vi "send response.vi"(6 "udp message":string, 7 "connection ID out":refnum<k16>, 8 "error in (no error)":errorcluster, 9 "port":u16, 10 "address":u32, 11 "command_parser in":refnum<class "command_parser.lvclass">) -> (0 "error out":errorcluster, 3 "command_parser out":refnum<class "command_parser.lvclass">)   [LabVIEW 2025, in "command_parser.lvlib" / "command_parser.lvclass"]
uses:
  command_parser.lvclass
  Applications/National Instruments/LabVIEW 2025 64-bit/vi.lib/ActorFramework/Actor/Actor.lvclass
  command_parser.lvclass/command_parser.ctl
  Send Notification Messages/send response Msg/send response Msg.lvclass/send response Msg.ctl
  <vilib>/ActorFramework/Message Enqueuer/Message Enqueuer.lvclass/Message Enqueuer.ctl
  <vilib>/ActorFramework/Actor/Actor.lvclass/Actor.ctl
  <vilib>/ActorFramework/Message Enqueuer/Enqueue.vi
  Send Notification Messages/send response Msg/send response Msg.lvclass
  Applications/National Instruments/LabVIEW 2025 64-bit/vi.lib/ActorFramework/Message/Message.lvclass
  <vilib>/ActorFramework/Stop Msg/Stop Msg.lvclass
  <vilib>/ActorFramework/Message Priority Queue/Priority Enqueue.vi
  <vilib>/ActorFramework/Actor/Actor.lvclass
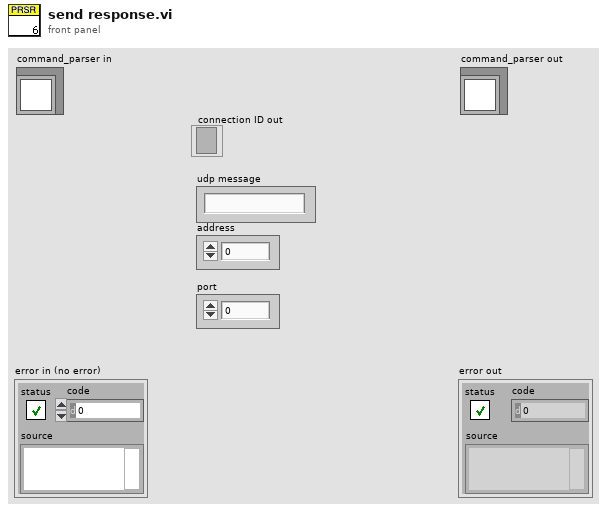
[diagram p1: front panel]
types:
  T1 = map{string, refnum<class "Message Enqueuer.lvclass">}
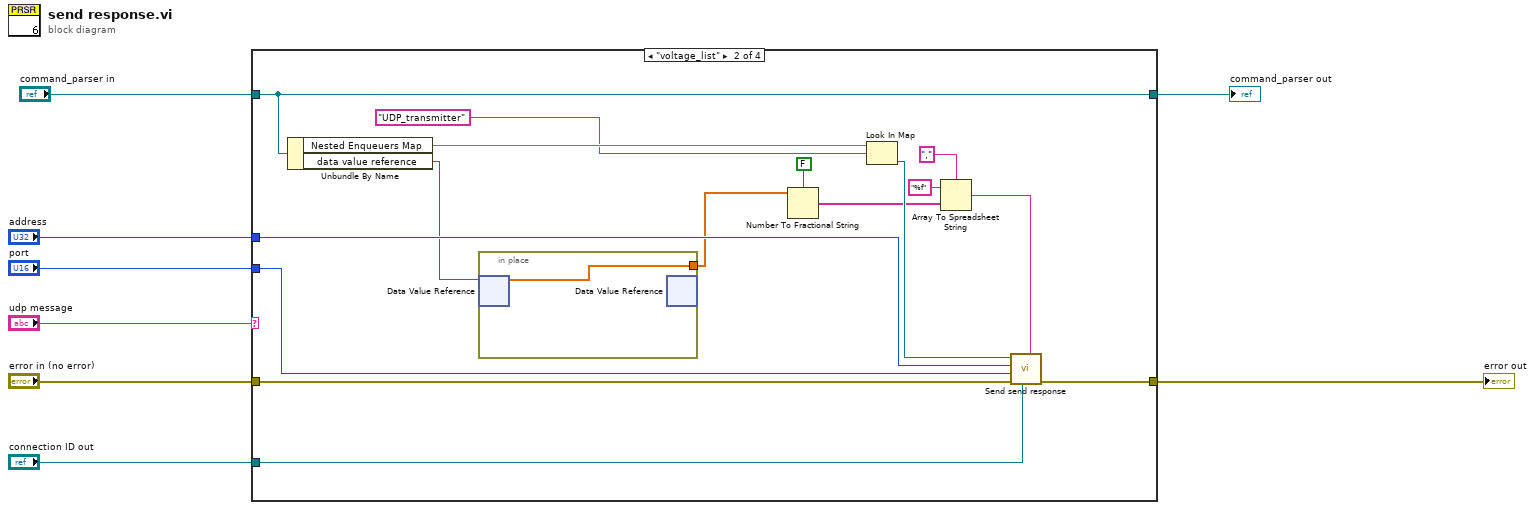
[diagram p0: block diagram]
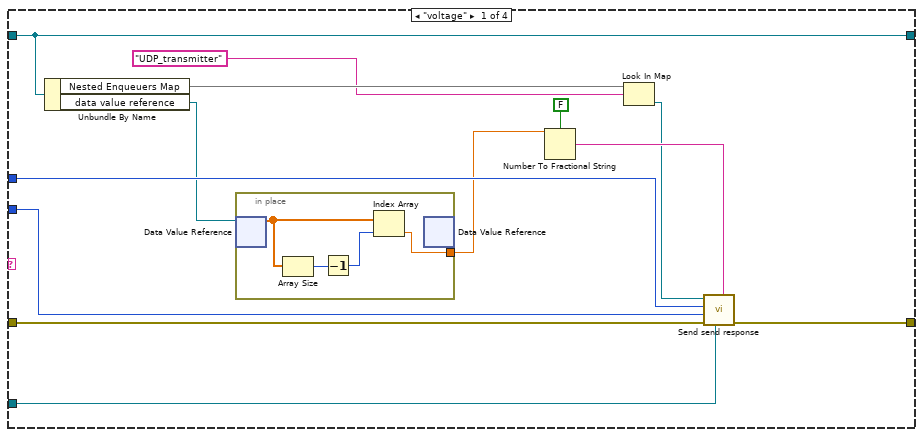
[diagram p2: hidden frame]
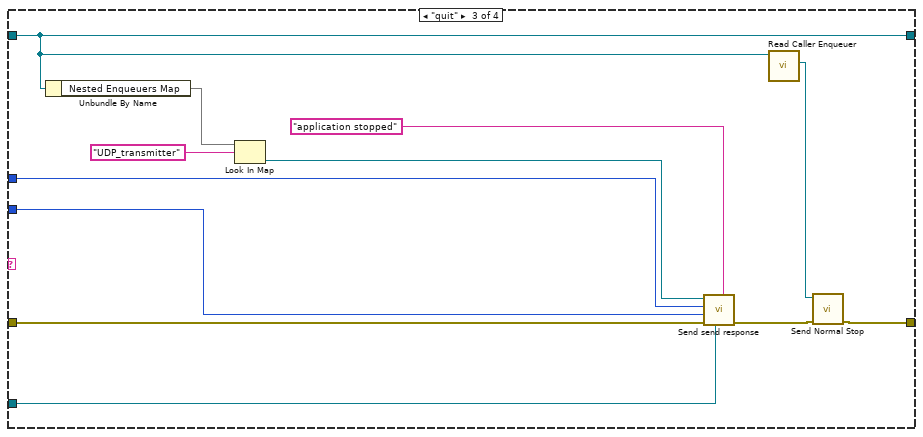
[diagram p3: hidden frame]
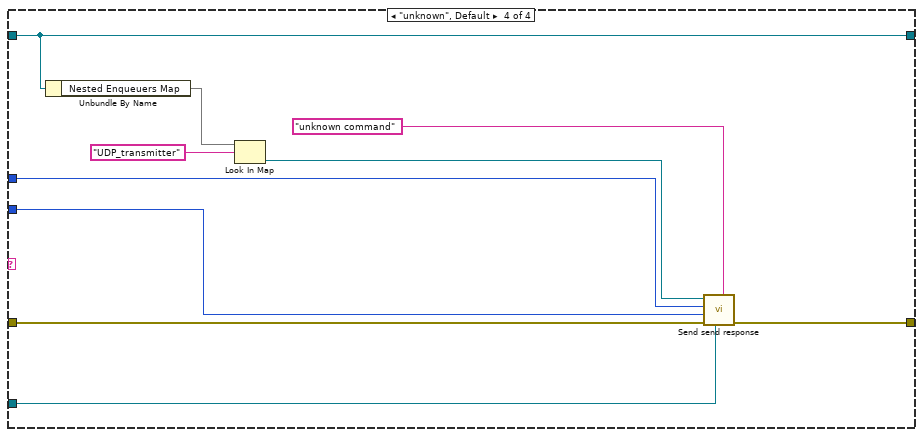
[diagram p4: hidden frame]
diagram:
  n1 = case shown="\"voltage_list\"" "udp message" {
    tunnel: "connection ID out" -> [w12 w33 w48 w58]
    tunnel: "address" -> [w14 w35 w50 w60]
    tunnel: "port" -> [w13 w34 w49 w59]
    tunnel: [w16 w37 w44 w55] -> w5
    tunnel: "error in (no error)" -> [w17 w38 w52 w62]
    tunnel: "command_parser in" -> [w19 w39 w43 w56]
    tunnel: [w19 w39 w43 w56] -> w1
    frame "voltage" {
      n2 = Unbundle By Name(w19) -> ("Nested Enqueuers Map"=w21:T1, "data value reference"=w11:refnum<data-value>)
      n3 = in-place {
        in-place-border: [w22] -> w10
        n4 = in-place-dvr #1(w11) -> (w23:dbl[])  [unwired: 1 out]
        n5 = Array Size(array=w23) -> (size(s)=w25:i32)
        n6 = Decrement(x=w25) -> (x-1=w24:i32)
        n7 = Index Array(array=w23, index=w24) -> (element=w22:dbl)
        n8 = in-place-dvr #1() -> ()  [unwired: 1 in, 2 out]
      }
      n9 = Number To Fractional String(use system decimal point (T)=FALSE, number=w10) -> (F-format string=w18:string)  [unwired: 2 in]
      n10 = Look In Map(map=w21, key="UDP_transmitter") -> (value=w15:refnum<class "Message Enqueuer.lvclass">)  [unwired: 1 in, 1 out]
      n11 = call "Send send response.vi"("udp message"=w18, "connection ID out"=w12, "error in (no error)"=w17, "port"=w13, "address"=w14, "Message Enqueuer"=w15) -> ("error out"=w16:errorcluster)  [unwired: 4 in, 1 out]
    }
    frame "voltage_list" {
      n12 = Unbundle By Name(w39) -> ("Nested Enqueuers Map"=w41:T1, "data value reference"=w32:refnum<data-value>)
      n13 = in-place {
        in-place-border: [w42] -> w30
        n14 = in-place-dvr #2(w32) -> (w42:dbl[])  [unwired: 1 out]
        n15 = in-place-dvr #2() -> ()  [unwired: 1 in, 2 out]
      }
      n16 = Number To Fractional String(use system decimal point (T)=FALSE, number=w30) -> (F-format string=w29:string[])  [unwired: 2 in]
      n17 = Look In Map(map=w41, key="UDP_transmitter") -> (value=w36:refnum<class "Message Enqueuer.lvclass">)  [unwired: 1 in, 1 out]
      n18 = Array To Spreadsheet String(delimiter (Tab)=",", array=w29, 3:"%f" ("format string")) -> (spreadsheet string=w27:string)
      n19 = call "Send send response.vi"("udp message"=w27, "connection ID out"=w33, "error in (no error)"=w38, "port"=w34, "address"=w35, "Message Enqueuer"=w36) -> ("error out"=w37:errorcluster)  [unwired: 4 in, 1 out]
    }
    frame "quit" {
      n20 = Unbundle By Name(w43) -> ("Nested Enqueuers Map"=w54:T1)
      n21 = Look In Map(map=w54, key="UDP_transmitter") -> (value=w51:refnum<class "Message Enqueuer.lvclass">)  [unwired: 1 in, 1 out]
      n22 = call "Send send response.vi"("udp message"="application stopped" ("data in"), "connection ID out"=w48, "error in (no error)"=w52, "port"=w49, "address"=w50, "Message Enqueuer"=w51) -> ("error out"=w45:errorcluster)  [unwired: 4 in, 1 out]
      n23 = call <vilib>:"Read Caller Enqueuer.vi"("Actor"=w43) -> ("Caller Enqueuer"=w46:refnum<class "Message Enqueuer.lvclass">)  [unwired: 10 in]
      n24 = call <vilib>:"Send Normal Stop.vi"("error in (no error)"=w45, "Message Enqueuer"=w46) -> ("error out"=w44:errorcluster)  [unwired: 9 in]
    }
    frame "unknown", Default {
      n25 = Unbundle By Name(w56) -> ("Nested Enqueuers Map"=w64:T1)
      n26 = Look In Map(map=w64, key="UDP_transmitter") -> (value=w61:refnum<class "Message Enqueuer.lvclass">)  [unwired: 1 in, 1 out]
      n27 = call "Send send response.vi"("udp message"="unknown command" ("data in"), "connection ID out"=w58, "error in (no error)"=w62, "port"=w59, "address"=w60, "Message Enqueuer"=w61) -> ("error out"=w55:errorcluster)  [unwired: 4 in, 1 out]
    }
  }
  "error out" <- w5
  "command_parser out" <- w1
